vi "onComputeIntervals.vi"(8 "error in (no error)":errorcluster, 9 "Cron Interval":T1, 10 "Expression":string, 11 "Cron.Unix in":refnum<class "Cron.Unix.lvclass">) -> (0 "error out":errorcluster, 2 "Interval Parameters":T2, 3 "Cron.Unix out":refnum<class "Cron.Unix.lvclass">)   [LabVIEW 2013, in "openCron.lvlib" / "Cron.Unix.lvclass"]
uses:
  Cron.Unix.lvclass
  Cron/Cron Interval -- cluster.ctl
  Cron/Cron Interval -- enum.ctl
  Cron/Cron.lvclass
panel:
  out "remaining string":string
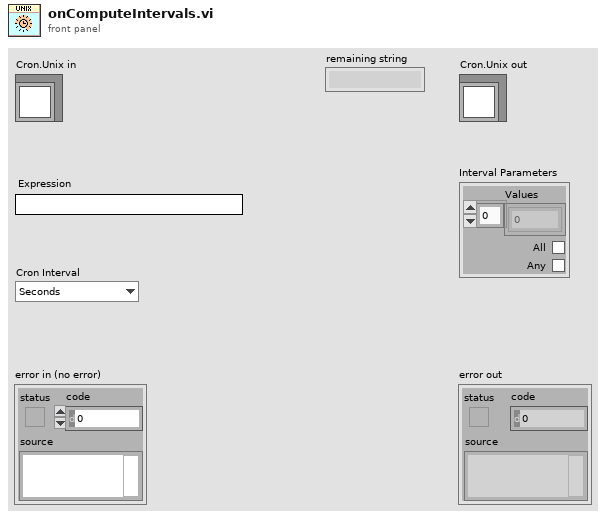
[diagram p1: front panel]
types:
  T1 = typedef "openCron.lvlib/Cron.lvclass/Cron Interval -- enum.ctl" = enum16{"Seconds", "Minutes", "Hours", "Day of Month", "Month", "Day of Week", "Year"}
  T2 = typedef "openCron.lvlib/Cron.lvclass/Cron Interval -- cluster.ctl" = cluster{"Values":i32[], "All":bool, "Any":bool}
  T3 = enum16{"SUN", "MON", "TUE", "WED", "THU", "FRI", "SAT"}
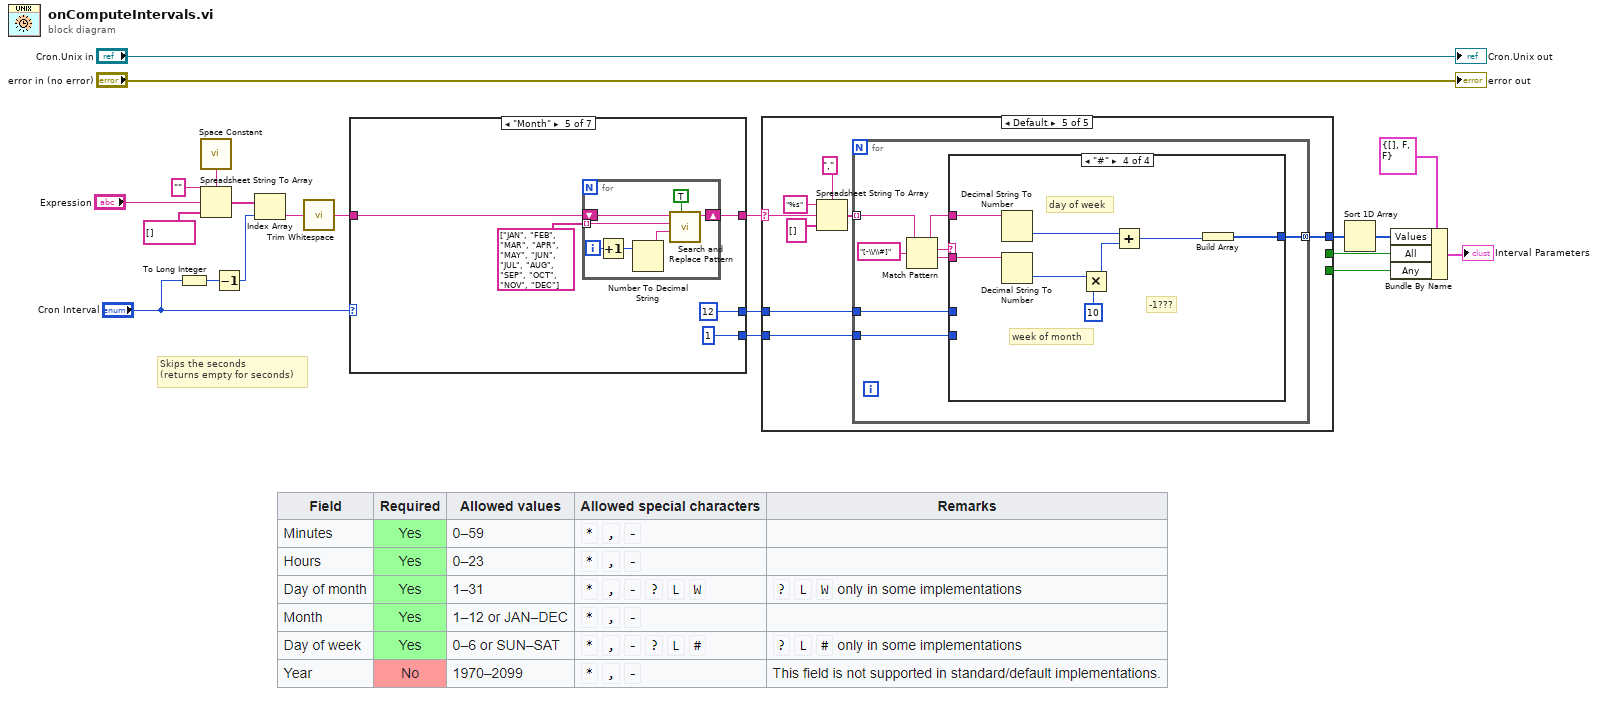
[diagram p0: block diagram]
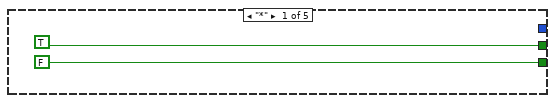
[diagram p2: hidden frame]
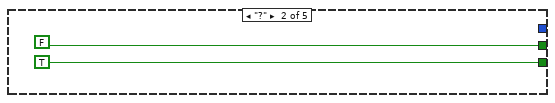
[diagram p3: hidden frame]
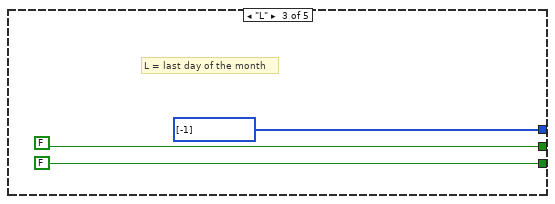
[diagram p4: hidden frame]
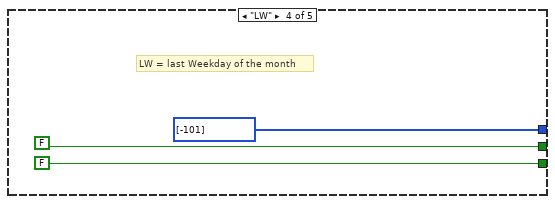
[diagram p5: hidden frame]
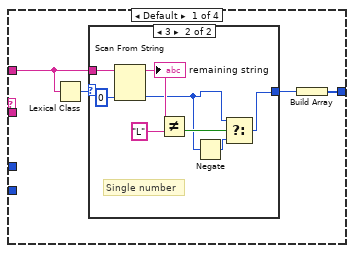
[diagram p6: hidden frame]
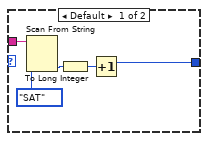
[diagram p7: hidden frame]
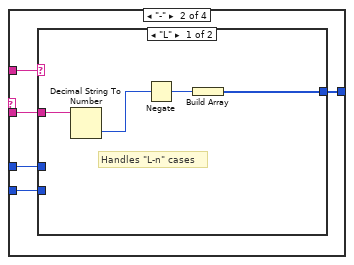
[diagram p8: hidden frame]
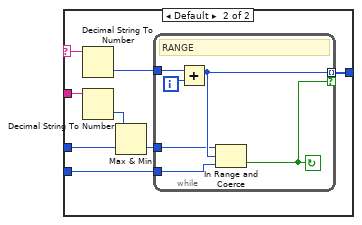
[diagram p9: hidden frame]
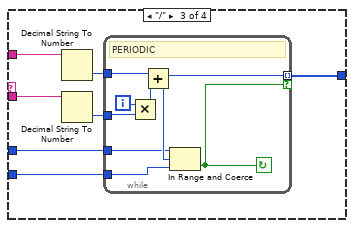
[diagram p10: hidden frame]
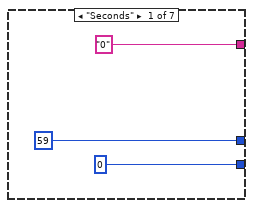
[diagram p11: hidden frame]
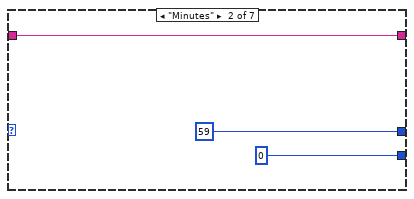
[diagram p12: hidden frame]
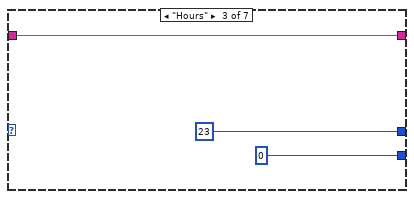
[diagram p13: hidden frame]
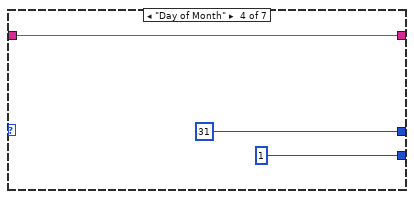
[diagram p14: hidden frame]
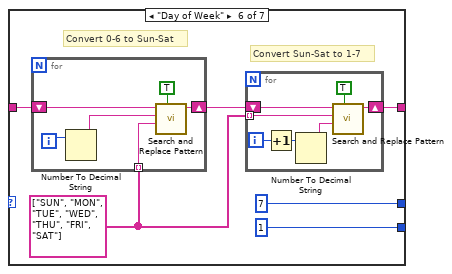
[diagram p15: hidden frame]
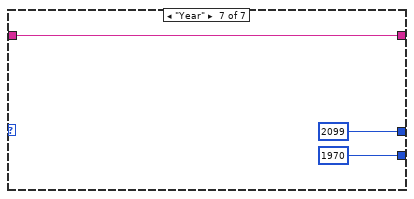
[diagram p16: hidden frame]
diagram:
  # "Skips the seconds\n(returns empty for seconds)"
  n1 = To Long Integer(number="Cron Interval") -> (32bit integer=w3:i32)
  n2 = call <vilib>:"Space Constant.vi"() -> ("String"=w16:string)
  n3 = Spreadsheet String To Array(delimiter (Tab)=w16, format string="", spreadsheet string="Expression", array type (2D Dbl)=string[] []) -> (array=w15:string[])
  n4 = Decrement(x=w3) -> (x-1=w1:i32)
  n5 = Index Array(array=w15, index=w1) -> (element=w13:string)
  n6 = call <vilib>:"Trim Whitespace.vi"("string"=w13) -> ("trimmed string"=w5:string)  [unwired: 1 in]
  n7 = case shown="\"Month\"" "Cron Interval" {
    tunnel: [59 ("y") 59 ("y") 23 ("y") 31 ("y") 12 ("y") 7 ("y") 2099 ("y")] -> w12
    tunnel: [0 ("y") 0 ("y") 0 ("y") 1 ("y") 1 ("y") 1 ("y") 1970 ("y")] -> w11
    tunnel: w5 -> [_ w25 w28 w31 w35 w48 w65]
    tunnel: ["0" ("trimmed string") w25 w28 w31 w36 w49 w65] -> w4
    frame "Seconds" {
    }
    frame "Minutes" {
    }
    frame "Hours" {
    }
    frame "Day of Month" {
    }
    frame "Month" {
      n8 = for {
        shift-right: [w45] -> w36
        shift-left: w35 -> [w44]
        tunnel: string[] ["JAN", "FEB", "MAR", "APR", "MAY", "JUN", "JUL", "AUG", "SEP", "OCT", "NOV", "DEC"] -> [w42] mode=indexing
        i -> [w41]
        n9 = Increment(x=w41) -> (x+1=w40:i32)
        n10 = Number To Decimal String(number=w40) -> (decimal integer string=w39:string)  [unwired: 1 in]
        n11 = call <vilib>:"Search and Replace Pattern.vi"("string"=w44, "regular expression (\"\")"=w42, "replace string (\"\")"=w39, "replace all? (F)"=TRUE) -> ("result string"=w45:string)  [unwired: 1 in, 1 out]
      }
    }
    frame "Day of Week" {
      w46 = string[] ["SUN", "MON", "TUE", "WED", "THU", "FRI", "SAT"]
      # "Convert Sun-Sat to 1-7"
      # "Convert 0-6 to Sun-Sat"
      n12 = for {
        shift-right: [w57] -> w47
        shift-left: w48 -> [w56]
        tunnel: w46 -> [w54] mode=indexing
        i -> [w53]
        n13 = Number To Decimal String(number=w53) -> (decimal integer string=w52:string)  [unwired: 1 in]
        n14 = call <vilib>:"Search and Replace Pattern.vi"("string"=w56, "regular expression (\"\")"=w52, "replace string (\"\")"=w54, "replace all? (F)"=TRUE) -> ("result string"=w57:string)  [unwired: 1 in, 1 out]
      }
      n15 = for {
        shift-right: [w64] -> w49
        shift-left: w47 -> [w63]
        tunnel: w46 -> [w61] mode=indexing
        i -> [w59]
        n16 = Increment(x=w59) -> (x+1=w58:i32)
        n17 = Number To Decimal String(number=w58) -> (decimal integer string=w60:string)  [unwired: 1 in]
        n18 = call <vilib>:"Search and Replace Pattern.vi"("string"=w63, "regular expression (\"\")"=w61, "replace string (\"\")"=w60, "replace all? (F)"=TRUE) -> ("result string"=w64:string)  [unwired: 1 in, 1 out]
      }
    }
    frame "Year" {
    }
  }
  n19 = case shown="Default" w4 {
    selector: w4 -> [_ _ _ _ w81]
    tunnel: [_ _ i32[] [-1] i32[] [-101] w80] -> w9
    tunnel: [TRUE FALSE FALSE FALSE _] -> w8
    tunnel: [FALSE TRUE FALSE FALSE _] -> w7
    tunnel: w12 -> [_ _ _ _ w79]
    tunnel: w11 -> [_ _ _ _ w78]
    frame "*" {
    }
    frame "?" {
    }
    frame "L" {
      # "L = last day of the month"
    }
    frame "LW" {
      # "LW = last Weekday of the month"
    }
    frame Default {
      n20 = Spreadsheet String To Array(delimiter (Tab)=",", format string="%s", spreadsheet string=w81, array type (2D Dbl)=string[] []) -> (array=w82:string[])
      n21 = for {
        tunnel: w82 -> [w93] mode=indexing
        tunnel: [w89] -> w80 mode=concatenating
        tunnel: w79 -> [w87]
        tunnel: w78 -> [w86]
        n22 = Match Pattern(string=w93, regular expression="[-\\/\\#]") -> (before substring=w90:string, match substring=w91:string, after substring=w88:string)  [unwired: 1 in, 1 out]
        n23 = case shown="\"#\"" w91 {
          tunnel: w90 -> [w95 w111 w140 w156]
          tunnel: [w96 w114 w138 w154] -> w89
          tunnel: w88 -> [_ w115 w136 w155]
          tunnel: w87 -> [_ w113 w135 _]
          tunnel: w86 -> [_ w112 w134 _]
          frame Default {
            n24 = Lexical Class(1:w95) -> (0:w94:i16)
            n25 = case shown="3" w94 {
              tunnel: [w98 w105] -> w97
              tunnel: w95 -> [w102 w110]
              frame Default {
                n26 = Scan From String(input string=w102, default 1=T3."SAT" ("y")) -> (output 1=w99:T3)  [unwired: 3 in, 3 out]
                n27 = To Long Integer(number=w99) -> (32bit integer=w100:i32)
                n28 = Increment(x=w100) -> (x+1=w98:i32)
              }
              frame 3 {
                # "Single number"
                n29 = Scan From String(input string=w110, default 1=0 ("number")) -> (remaining string=w108:string, output 1=w104:i32)  [unwired: 3 in, 2 out]
                "remaining string" <- w108
                n30 = Not Equal?(x=w108, y="L") -> (x != y?=w106:bool)
                n31 = Negate(x=w104) -> (-x=w103:i32)
                n32 = Select(t=w104, s=w106, f=w103) -> (s? t:f=w105:i32)
              }
            }
            n33 = Build Array(w97) -> (w96:i32[])
          }
          frame "-" {
            n34 = case shown="\"L\"" w111 {
              selector: w111 -> [_ w120]
              tunnel: w115 -> [w119 w126]
              tunnel: [w117 w125] -> w114
              tunnel: w113 -> [_ w123]
              tunnel: w112 -> [_ w122]
              frame "L" {
                # "Handles \"L-n\" cases"
                n35 = Decimal String To Number(string=w119) -> (number=w118:i32)  [unwired: 2 in, 1 out]
                n36 = Negate(x=w118) -> (-x=w116:i32)
                n37 = Build Array(w116) -> (w117:i32[])
              }
              frame Default {
                n38 = Decimal String To Number(string=w120) -> (number=w127:i32)  [unwired: 2 in, 1 out]
                n39 = Decimal String To Number(string=w126) -> (number=w124:i32)  [unwired: 2 in, 1 out]
                n40 = Max & Min(x=w124, y=w123) -> (min(x,y)=w121:i32)  [unwired: 1 out]
                n41 = while {
                  tunnel: w127 -> [w133]
                  tunnel: [w130] -> w125 mode=indexing if=w131
                  tunnel: w122 -> [w129]
                  tunnel: w121 -> [w128]
                  i -> [w132]
                  stop <- w131 continue-if-true
                  # "RANGE"
                  n42 = Add(x=w133, y=w132) -> (x+y=w130:i32)
                  n43 = In Range and Coerce(upper limit=w128, x=w130, lower limit=w129) -> (In Range?=w131:bool)  [unwired: 1 out]
                }
              }
            }
          }
          frame "/" {
            n44 = Decimal String To Number(string=w140) -> (number=w139:i32)  [unwired: 2 in, 1 out]
            n45 = Decimal String To Number(string=w136) -> (number=w137:i32)  [unwired: 2 in, 1 out]
            n46 = while {
              tunnel: w139 -> [w148]
              tunnel: [w144] -> w138 mode=indexing if=w141
              tunnel: w137 -> [w147]
              tunnel: w135 -> [w143]
              tunnel: w134 -> [w142]
              i -> [w146]
              stop <- w141 continue-if-true
              # "PERIODIC"
              n47 = Multiply(x=w146, y=w147) -> (x*y=w145:i32)
              n48 = Add(x=w148, y=w145) -> (x+y=w144:i32)
              n49 = In Range and Coerce(upper limit=w143, x=w144, lower limit=w142) -> (In Range?=w141:bool)  [unwired: 1 out]
            }
          }
          frame "#" {
            # "-1???"
            # "week of month"
            # "day of week"
            n50 = Decimal String To Number(string=w156) -> (number=w149:i32)  [unwired: 2 in, 1 out]
            n51 = Decimal String To Number(string=w155) -> (number=w153:i32)  [unwired: 2 in, 1 out]
            n52 = Multiply(x=w153, y=10) -> (x*y=w151:i32)
            n53 = Add(x=w149, y=w151) -> (x+y=w150:i32)
            n54 = Build Array(w150) -> (w154:i32[])
          }
        }
      }
    }
  }
  n55 = Sort 1D Array(array=w9) -> (sorted array=w10:i32[])
  n56 = Bundle By Name(cluster=T2 {"Values"=[], "All"=FALSE, "Any"=FALSE} ("Interval"), "Values"=w10, "All"=w8, "Any"=w7) -> (→"Interval Parameters":T2)
  "error out" <- "error in (no error)"
  "Cron.Unix out" <- "Cron.Unix in"
